vi "ReadBinaryWaveformFile old.vi"(8 "error in (no error)":errorcluster, 9 "start of read offset (bytes:0)":i32, 11 "file path (dialog if empty)":path) -> (0 "error out":errorcluster, 1 "1D array":sgl[](array[numeric]) format="%.3f", 2 "2D array":sgl[][](array[numeric]) format="%.3f", 3 "new file path (Not A Path if cancelled)":path, 4 "EOF?":bool, 5 "mark after read (bytes)":i32, 6 "Time base":dbl format="%.6e", 7 "Delay, points":dbl format="%.2f")   [LabVIEW 2021]
doc: "Reads a 2D or 1D array of data from a byte stream file of single-precision numbers (SGL). The VI opens the file beforehand and closes it afterwards. You can use this VI to read scaled data acquired from data acquisition VIs and written to a file with Write To SGL File.\n\nfile path is the path name of the file. If file path is empty (default value) or is Not A Path, the VI displays a File dialog box from which you can select a file. Error 43 occurs if the user cancels the dialog. \n\n¥ To read the entire file into 1D array, set 1D count <0 (default); you can leave 2D number of rows unwired.\n¥ To read N elements into 1D array, set 1D count =N and leave 2D number of rows wired or set to 0.\n¥ To read the entire file into 2D array, set 2D number of rows <0 and 2D number of columns =N >0. The VI calculates the number of rows as the integer part of file size/N.\n¥ To read M rows and N columns into 2D array, set 2D number of rows =M and 2D number of columns =N.\n\nstart of read offset is the position in the file, measured in bytes, at which the VI begins reading.\n\nnew file path is the path of the file from which the VI read data. You can use this output to determine the path of a file that you open using dialog. new file path returns Not A Path if the user selects Cancel from the dialog box.\n\n2D array contains the single precision numbers read from the file if 2D number of columns is >0 and 2D number of rows is <0 (meaning read the entire file) or >0 (read the the specified number of rows) ; otherwise, this output is empty.\n\n1D array contains the single precision numbers read from the file if 1D count is <0 (meaning read the entire file) or 2D number of rows =0 and 1D count is >0 (meaning read the specified number of samples); otherwise, this output is empty.\n\nmark after read is the location of the file mark after the read; it points to the byte in the file following the last byte read.\n\nEOF? is TRUE if you attempt to read past the end of file.\n\nRevisions:\n21 Oct 93: changes incorporated to read entire file (default to read entire file as 1D array); cosmetic changes.\n12 May 94: documentation changes."
panel:
  out "2D number of rows":i32
  out "2D number of columns/1D count":i32
  in  "prompt":string="Choose file to read."
  in  "instructions":string="* To read the entire file into 1D array, set 1D count <0 (default); you can leave 2D number of rows unwired.\n* To read N elements into 1D array, set 1D count =N and leave 2D number of rows wired or set to 0.\n* To read the entire file into 2D array, set 2D number of rows <0 and 2D number of columns =N >0.  The VI calculates the number of rows as the integer part of file size/N.\n* To read M rows and N columns into 2D array, set 2D number of rows =M and 2D number of columns =N."
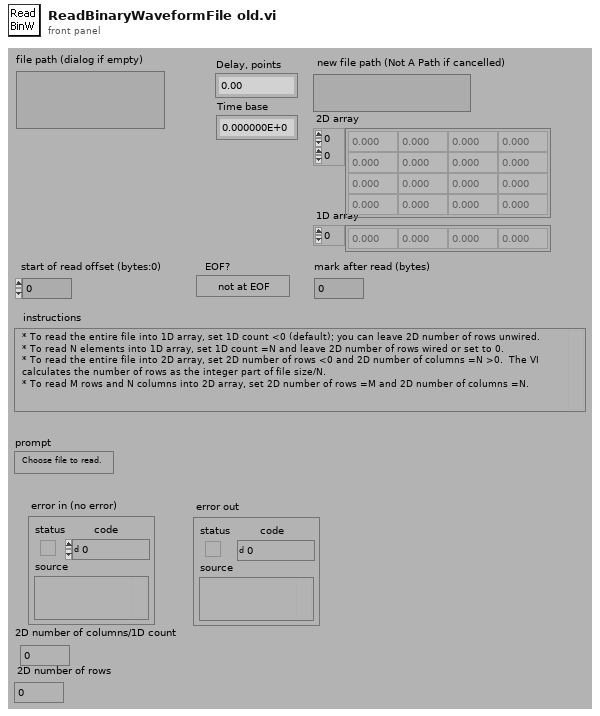
[diagram p1: front panel]
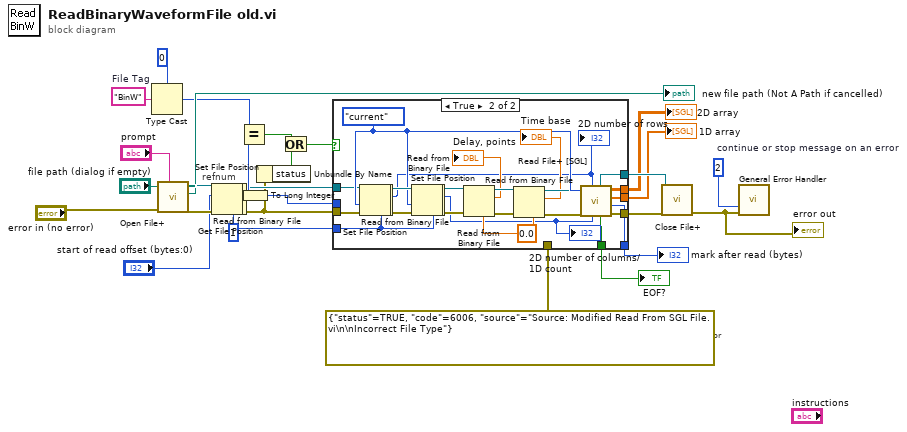
[diagram p0: block diagram]
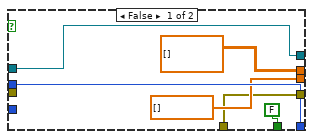
[diagram p2: hidden frame]
diagram:
  w12 = "BinW"  # File Tag
  w18 = 1 ("count")
  w31 = u16 2  # continue or stop message on an error
  # "error"
  # "refnum"
  n1 = Type Cast(type=0, x=w12) -> (*(type *) &x=w10:i32)
  n2 = call <vilib>:"Open File+.vi"("prompt"="prompt", "error in (not an error)"="error in (no error)", "file path (\" \")"="file path (dialog if empty)") -> ("error out"=w21:errorcluster, "file path"=→"new file path (Not A Path if cancelled)":path, "refnum"=w22:refnum<file>)  [unwired: 3 in, 3 out]
  n3 = Set File Position(offset (in bytes) (0)="start of read offset (bytes:0)", refnum=w22, error in=w21) -> (refnum out=w5:refnum<file>, error out=w4:errorcluster)  [unwired: 1 out]
  n4 = Read from Binary File(5:w18, 8:w4, 11:w5) -> (0:w2:errorcluster, 2:w20:i32, 3:w3:refnum<file>)  [unwired: 4 out]
  n5 = Get File Position(4:w2, 7:w3) -> (0:w9:errorcluster, 2:w1:i64, 3:w19:refnum<file>)
  n6 = Equal?(x=w10, y=w20) -> (x = y?=w7:bool)
  n7 = To Long Integer(number=w1) -> (32bit integer=w16:i32)
  n8 = Unbundle By Name(w9) -> ("status"=w8:bool)
  n9 = Or(x=w7, y=w8) -> (x .or. y?=w6:bool)
  n10 = case shown="True" w6 {
    tunnel: [w33 w65] -> w30
    tunnel: [w38 w64] -> w29
    tunnel: [FALSE ("EOF?") w63] -> w28
    tunnel: [w34 w62] -> w27
    tunnel: [sgl[] [] ("1D data") w61] -> w26
    tunnel: [sgl[][] [] ("2D data") w60] -> w25
    tunnel: w19 -> [w34 w56]
    tunnel: w9 -> [_ w55]
    tunnel: w18 -> [_ w45]
    tunnel: w16 -> [w38 _]
    tunnel: errorcluster {"status"=TRUE, "code"=6006, "source"="Source: Modified Read From SGL File.vi\n\nIncorrect File Type"} ("error out") -> [w33 _]
    frame False {
    }
    frame True {
      w46 = 0.0
      w57 = enum16{"start", "end", "current"}."current" ("pos mode (0:2)")
      n11 = Set File Position(refnum=w56, from (0:start)=w57, error in=w55) -> (refnum out=w40:refnum<file>, error out=w39:errorcluster)  [unwired: 1 out]
      n12 = Read from Binary File(5:w45, 8:w39, 11:w40) -> (0:w59:errorcluster, 2:w43:i32, 3:w58:refnum<file>)  [unwired: 4 out]
      "2D number of rows" <- w43
      n13 = Set File Position(refnum=w58, from (0:start)=w57, error in=w59) -> (refnum out=w42:refnum<file>, error out=w41:errorcluster)  [unwired: 1 out]
      n14 = Read from Binary File(5:w45, 8:w41, 11:w42) -> (0:w51:errorcluster, 2:w44:i32, 3:w54:refnum<file>)  [unwired: 4 out]
      "2D number of columns/1D count" <- w44
      n15 = Read from Binary File(5:w46, 8:w51, 11:w54) -> (0:w50:errorcluster, 2:→"Delay, points":dbl, 3:w53:refnum<file>)  [unwired: 4 out]
      n16 = Read from Binary File(5:w46, 8:w50, 11:w53) -> (0:w49:errorcluster, 2:→"Time base":dbl, 3:w52:refnum<file>)  [unwired: 4 out]
      n17 = call <vilib>:"Read File+ [SGL].vi"("2D number of columns/1D count"=w44, "2D number of rows"=w43, "error in (no error)"=w49, "pos mode (rel. to current:2)"=w57, "refnum"=w52) -> ("error out"=w65:errorcluster, "mark after read (bytes)"=w64:i32, "1D data"=w61:sgl[], "2D data"=w60:sgl[][], "EOF?"=w63:bool, "dup refnum"=w62:refnum<file>)  [unwired: 1 in]
    }
  }
  "1D array" <- w26
  "mark after read (bytes)" <- w29
  "EOF?" <- w28
  "2D array" <- w25
  n18 = call <vilib>:"Close File+.vi"("error in (no error)"=w30, "refnum"=w27) -> ("error out"=w13:errorcluster)  [unwired: 5 out]
  "error out" <- w13
  n19 = call <vilib>:"General Error Handler.vi"("type of dialog (OK msg:1)"=w31, "error in (no error)"=w13) -> ()  [unwired: 1 in, 13 out]
